vi "HGF_DFSMVisitor.appendData2Variant.vi"(0 "initData":variant, 2 "trigger":T1=enum."visit", 3 "deviceVisitor":refnum<class "HGF_DeviceVisitor.lvclass">, 5 "error in (no error)":errorcluster) -> (14 "dup initData":variant, 19 "error out":errorcluster)   [LabVIEW 2012, in "HGF_DeviceFSM.lvlib" / "HGF_DFSMVisitor.lvclass"]
uses:
  HGF_DFSMVisitor.lvclass
  HGF_DeviceBaseClasses/HGF_DeviceVisitor/HGF_DeviceVisitor.lvclass
  HGF_DeviceFSM/HGF_DeviceFSM.lvsc/Trigger.ctl
  HGF_DeviceFSM/HGF_DeviceFSM.lvsc
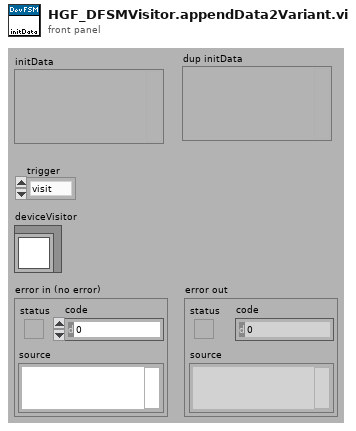
[diagram p1: front panel]
types:
  T1 = typedef "HGF_DeviceFSM.lvlib/HGF_DeviceFSM.lvsc/Trigger.ctl" = enum16{"NULL", "configure", "fault", "error", "resetError", "STOP", "visit", "not_configured", "done", "ok", "previsit", "configured"}
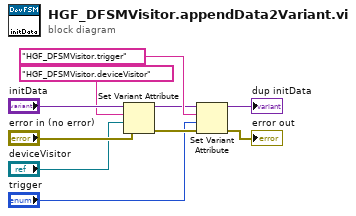
[diagram p0: block diagram]
diagram:
  n1 = Set Variant Attribute(Variant="initData", name="HGF_DFSMVisitor.deviceVisitor", value="deviceVisitor", error in="error in (no error)") -> (Variant out=w6:variant, error out=w7:errorcluster)  [unwired: 1 out]
  n2 = Set Variant Attribute(Variant=w6, name="HGF_DFSMVisitor.trigger", value="trigger", error in=w7) -> (Variant out=→"dup initData":variant, error out=→"error out":errorcluster)  [unwired: 1 out]
